vi "SLL DE DAQ LV2 Global.vi"(6 "Status Array In":bool[](array[boolean]), 7 "Option":T2, 8 "error in (no error)":errorcluster, 9 "Status In":bool, 10 "Elements Array":T1[](array[typedef]), 11 "Element":T1) -> (0 "error out":errorcluster, 2 "Status Array Out":bool[](array[boolean]), 3 "Status Out":bool)   [LabVIEW 2009]
uses:
  Sub VIs/DAQ Engine/Controls/SLL DE DAQ Global Options.ctl
  Sub VIs/DAQ Engine/Controls/SLL DE DAQ Global Elements.ctl
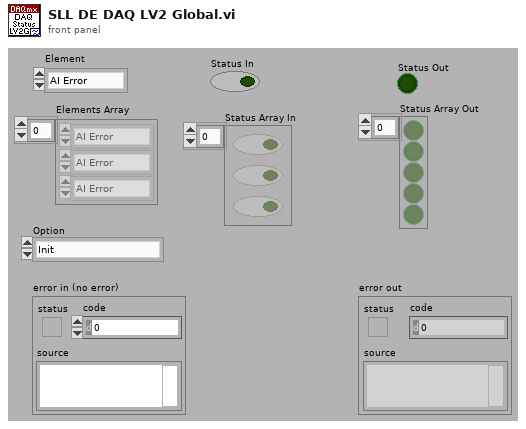
[diagram p1: front panel]
types:
  T1 = typedef "SLL DE DAQ Global Elements.ctl" = enum16{"AI Error", "AO Error", "DI Error", "DO Error", "AI Restart", "DI Restart", "AI Running", "AO Running", "DI Running", "DO Running", "DAQ Exit?"}
  T2 = typedef "SLL DE DAQ Global Options.ctl" = enum16{"Init", "Write 1", "Read 1", "Write Array", "Read Array", "Clear"}
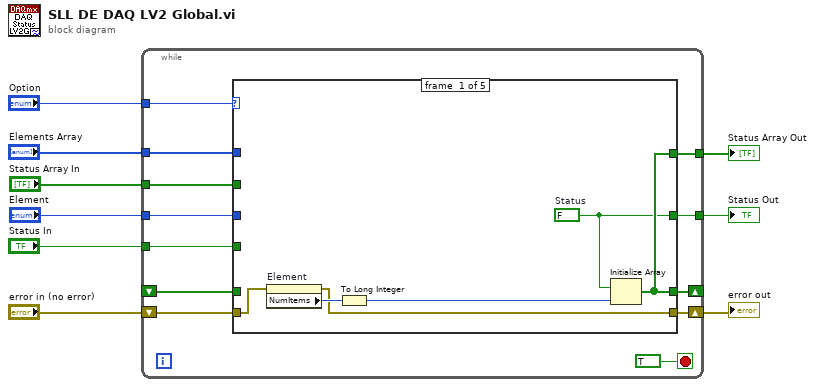
[diagram p0: block diagram]
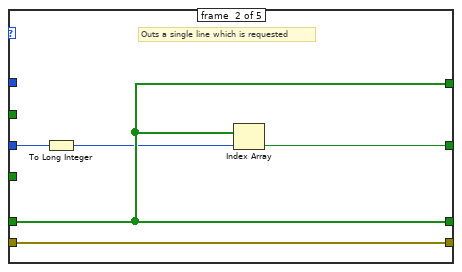
[diagram p2: hidden frame]
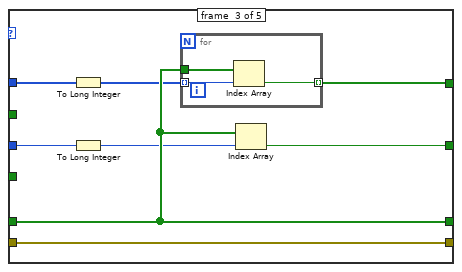
[diagram p3: hidden frame]
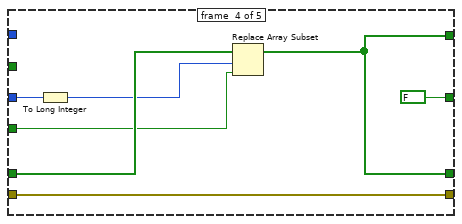
[diagram p4: hidden frame]
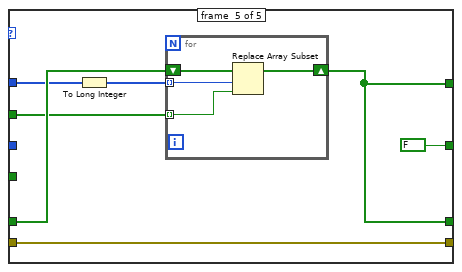
[diagram p5: hidden frame]
diagram:
  n1 = while {
    shift-right: [w20] -> _
    shift-left: _ -> [w19]
    tunnel: "Elements Array" -> [w18]
    tunnel: "Element" -> [w17]
    tunnel: [w16] -> w7
    tunnel: [w15] -> w6
    shift-right: [w13] -> w4
    shift-left: "error in (no error)" -> [w14]
    tunnel: "Status Array In" -> [w12]
    tunnel: "Status In" -> [w11]
    tunnel: "Option" -> [w10]
    stop <- TRUE stop-if-true
    n2 = case shown="\"Write 1\"" w10 {
      tunnel: [w27 w30 w37 w50 w57] -> w20
      tunnel: w19 -> [_ w30 w37 w47 w54]
      tunnel: w18 -> [_ _ w40 _ w52]
      tunnel: w17 -> [_ w32 w36 w45 _]
      tunnel: [w26 w31 w35 FALSE ("Digital Input") FALSE ("Digital Input")] -> w16
      tunnel: [w27 w30 w39 w50 w57] -> w15
      tunnel: w14 -> [w24 w29 w38 w48 w55]
      tunnel: [w23 w29 w38 w48 w55] -> w13
      tunnel: w12 -> [_ _ _ _ w53]
      tunnel: w11 -> [_ _ _ w46 _]
      frame #0 {
        w26 = FALSE  # Status
        n3 = property on="Element" class="Enum (strict)"(error in=w24) -> (error out=w23:errorcluster, "NumItems"=w25:u32)  [unwired: 1 in, 1 out]
        n4 = To Long Integer(number=w25) -> (32bit integer=w22:i32)
        n5 = Initialize Array(w26, w22) -> (w27:bool[])
      }
      frame #1 {
        # "Outs a single line which is requested"
        n6 = To Long Integer(number=w32) -> (32bit integer=w28:i32)
        n7 = Index Array(array=w30, index=w28) -> (element=w31:bool)
      }
      frame #2 {
        n8 = To Long Integer(number=w40) -> (32bit integer=w33:i32[])
        n9 = To Long Integer(number=w36) -> (32bit integer=w34:i32)
        n10 = for {
          tunnel: w37 -> [w43]
          tunnel: w33 -> [w42] mode=indexing
          tunnel: [w41] -> w39 mode=indexing
          n11 = Index Array(array=w43, index=w42) -> (element=w41:bool)
        }
        n12 = Index Array(array=w37, index=w34) -> (element=w35:bool)
      }
      frame #3 {
        n13 = To Long Integer(number=w45) -> (32bit integer=w44:i32)
        n14 = Replace Array Subset(array=w47, new element=w46, index=w44) -> (w50:bool[])
      }
      frame #4 {
        n15 = To Long Integer(number=w52) -> (32bit integer=w51:i32[])
        n16 = for {
          tunnel: w53 -> [w59] mode=indexing
          shift-right: [w60] -> w57
          shift-left: w54 -> [w61]
          tunnel: w51 -> [w58] mode=indexing
          n17 = Replace Array Subset(array=w61, new element=w59, index=w58) -> (w60:bool[])
        }
      }
    }
  }
  "error out" <- w4
  "Status Out" <- w7
  "Status Array Out" <- w6
